vi "monthFormatterSubVI.vi"(1 "month string in":string) -> (0 "month string out":string)   [LabVIEW 2011]
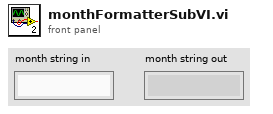
[diagram p1: front panel]
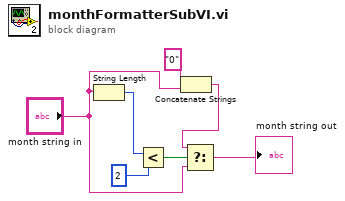
[diagram p0: block diagram]
diagram:
  n1 = String Length(string="month string in") -> (length=w1:i32)
  n2 = Less?(x=w1, y=2) -> (x < y?=w3:bool)
  n3 = Concatenate Strings("0" ("string"), "month string in") -> (w6:string)
  n4 = Select(t=w6, s=w3, f="month string in") -> (s? t:f=→"month string out":string)
